vi "Untitled 2.vi"   [LabVIEW 2010]
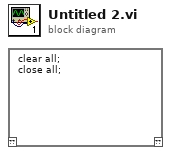
[diagram p0: block diagram]
diagram:
  n1 = script code="clear all;\nclose all;"() -> ()  [unwired: 1 in, 1 out]
